vi "CH_LM Wait for Service Request.vi"(0 "Meter Index":i32, 5 "error in (no error)":errorcluster, 7 "Timeout / ms (1000)":i32=1000) -> (13 "timed out?":bool, 14 "Meter Index":i32, 16 "Data String":string, 19 "error out":errorcluster)   [LabVIEW 2017, in "CH_LM.lvlib"]
doc: "Out-going Service Requests will be issued in order to provide a means of asynchronous communication over the IEEE-488 bus. The meter will assert the Service Request hardware line (SRQ) to indicate that data or error information is available to be read (specifically, when either the measurement data or error queues transition from empty to non-empty). Available data will be either measurement data records (see section 4.8.1) or error records (see section 4.6). \n\nWhen the host senses the assertion of SRQ, it will use a serial poll of the Status Byte Register (STB) for each device on the bus to determine the device requesting the service. The currently polled device is requesting service if bit 6 of the STB register is set. When the host discovers that the meter is requesting service, it must issue the appropriate commands to determine the type of records that are available to be read.\n\n<B>Attention:</B> This VI is intentionally reentrant!"
uses:
  CH_LM.lvlib
  _CH_LM/CH_LM Action Enumeration.ctl
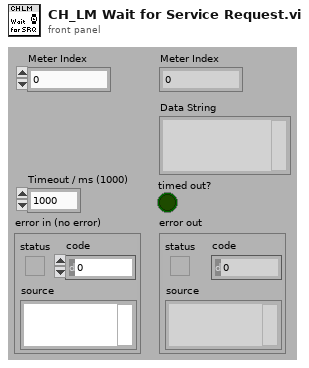
[diagram p1: front panel]
types:
  T1 = typedef "CH_LM.lvlib/CH_LM Action Enumeration.ctl" = enum16{"add", "read", "read by serial", "set", "remove", "delete", "Clear Shift-Register", ""}
  T2 = typedef "CH_LM.lvlib/CH_LM Meter Info.ctl" = cluster{"Meter Index":i32, "Serial Number":string, "Queue Cluster":T3, "Data Header":bool, "Data Tokens":T4[]}
  T3 = typedef "CH_LM.lvlib/CH_LM Queue Cluster.ctl" = cluster{"Streaming Queue":refnum<queue>, "Asynch Notifier":refnum<notifier>}
  T4 = typedef "CH_LM.lvlib/CH_LM Data Token.ctl" = enum16{"Raw data", "Quad distance", "Formated data", "Unit", "Pulse period", "Flags", "Sequence ID"}
  T5 = typedef "CH_LM.lvlib/CH_LM Event Cluster.ctl" = cluster{"Event Name":string, "Meter Index":i32, "Serial  Number":string, "Data":string, "iStreamingPacket":variant}
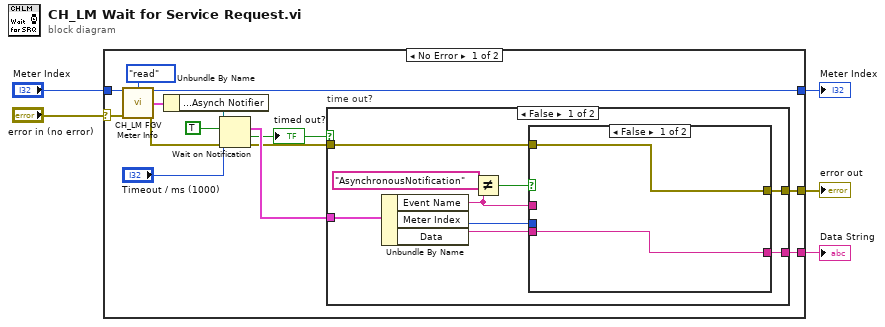
[diagram p0: block diagram]
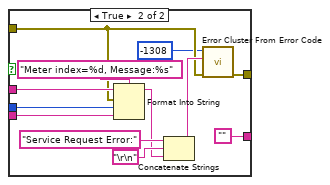
[diagram p2: hidden frame]
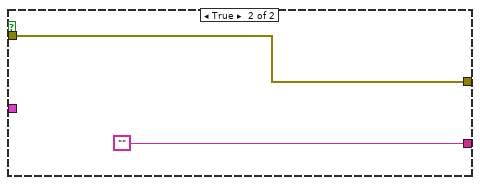
[diagram p3: hidden frame]
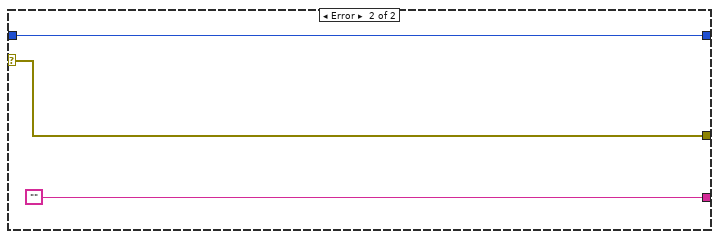
[diagram p4: hidden frame]
diagram:
  n1 = case shown="No Error" "error in (no error)" {
    selector: "error in (no error)" -> [w13 w47]
    tunnel: [w11 w47] -> w5
    tunnel: "Meter Index" -> [w12 w46]
    tunnel: [w8 w46] -> w2
    tunnel: [w7 ""] -> w1
    frame No Error {
      n2 = call "CH_LM FGV Meter Info.vi"("Meter Index"=w12, "Action (read)"=CH_LM_Action_Enumeration."read", "error in (no error)"=w13) -> ("Meter Index out"=w8:i32, "Meter Info"=w18:T2, "error out"=w15:errorcluster)  [unwired: 2 in, 8 out]
      n3 = Unbundle By Name(w18) -> ("Queue Cluster.Asynch Notifier"=w16:refnum<notifier>)
      n4 = Wait on Notification(notifier=w16, ignore previous (F)=TRUE, timeout in ms (-1)="Timeout / ms (1000)", error in (no error)=w15) -> (notification=w17:T5, timed out?=w9:bool, error out=w10:errorcluster)  [unwired: 1 out]
      "timed out?" <- w9
      n5 = case "time out?" shown="False" w9 {
        tunnel: w17 -> [w21 _]
        tunnel: [w23 w44] -> w11
        tunnel: w10 -> [w24 w44]
        tunnel: [w22 ""] -> w7
        frame False {
          n6 = Unbundle By Name(w21) -> ("Event Name"=w27:string, "Meter Index"=w26:i32, "Data"=w25:string)
          n7 = Not Equal?(x="AsynchronousNotification", y=w27) -> (x != y?=w20:bool)
          n8 = case shown="False" w20 {
            tunnel: w27 -> [_ w42]
            tunnel: w26 -> [_ w41]
            tunnel: w25 -> [w29 w40]
            tunnel: w24 -> [w30 w34]
            tunnel: [w30 w33] -> w23
            tunnel: [w29 ""] -> w22
            frame False {
            }
            frame True {
              n9 = Format Into String(format string="Meter index=%d, Message:%s", initial string=w42, error in=w34, w41, w40) -> (resulting string=w36:string)  [unwired: 1 out]
              n10 = Concatenate Strings("Service Request Error:" ("error message (\"\")"), "\r\n", w36) -> (w35:string)
              n11 = call <vilib>:"Error Cluster From Error Code.vi"("error in (no error)"=w34, "error message (\"\")"=w35, "error code (0)"=-1308) -> ("error out"=w33:errorcluster)  [unwired: 1 in, 5 out]
            }
          }
        }
        frame True {
        }
      }
    }
    frame Error {
    }
  }
  "error out" <- w5
  "Meter Index" <- w2
  "Data String" <- w1
